vi "transferData2UnitFormat.vi"(5 "Data":T1[](array[typedef])) -> (2 "display":dbl[][](array[numeric]))   [LabVIEW 2010]
uses:
  OutputDataFormat.ctl
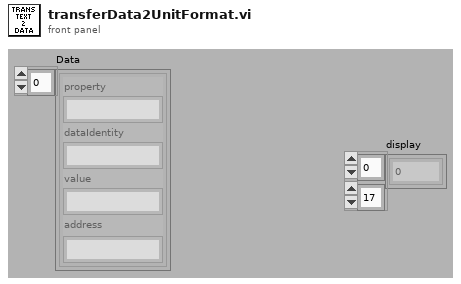
[diagram p1: front panel]
types:
  T1 = typedef "OutputDataFormat.ctl" = cluster{"property":string, "dataIdentity":string, "value":string, "address":string}
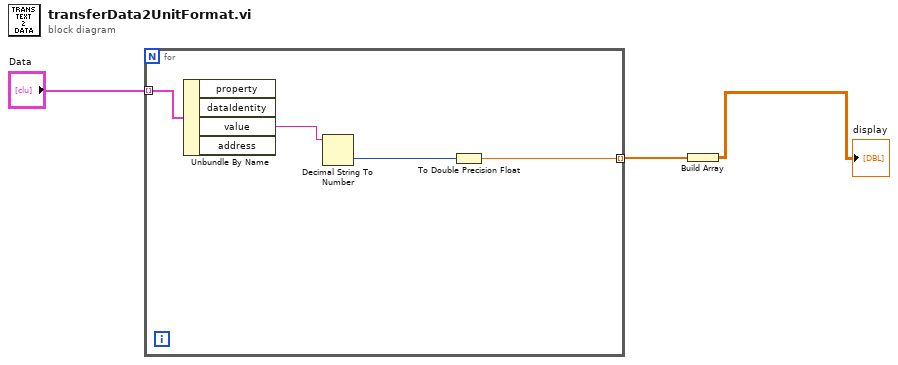
[diagram p0: block diagram]
diagram:
  n1 = for {
    tunnel: "Data" -> [w7] mode=indexing
    tunnel: [w5] -> w2 mode=indexing
    n2 = Unbundle By Name(w7) -> ("value"=w6:string)  [unwired: 3 out]
    n3 = Decimal String To Number(string=w6) -> (number=w4:i32)  [unwired: 2 in, 1 out]
    n4 = To Double Precision Float(number=w4) -> (double precision float=w5:dbl)
  }
  n5 = Build Array(w2) -> (→"display":dbl[][])
